vi "DCDC_Command.vi"(8 "error in (no error)":errorcluster, 9 "State":bool, 10 "Function Choose":T1, 11 "VISA resource in":refnum<visa-resource-name>="COM9") -> (0 "error out":errorcluster, 1 "Result":bool, 2 "read buffer":string, 3 "VISA resource out":refnum<visa-resource-name>)   [LabVIEW 2020]
uses:
  subvi/DCDC_Command.ctl
  ed6a49d5-09bc-4943-8c1b-6836990d678a.vi
  932ad59c-eb7e-44d9-8b1f-b581c4131119.vi
  c181c2eb-5caa-41f7-8f1d-9b0969fe7b32.vi
  9037c64f-12a5-4f95-b925-5e25449c8f50.vi
  f13df80e-a96c-4ee4-8010-69a0a001d2db.vi
  470163fb-24ed-4801-9874-fb3a4beeb085.vi
  c287b82f-2120-49b1-88be-16a92ee30e73.vi
  f2adf25f-970b-415f-a032-e0fcf203b769.vi
  9be719b3-8aa6-4acf-ac95-30d0a9685e01.vi
  5b62b920-1295-4d0c-95f0-4be6a500b32e.vi
  654ba534-6598-400c-ba18-c9c01572c5a6.vi
  4029cff3-6ee8-466a-8162-b4f2fed149be.vi
  8d00504a-0fe9-4555-a6c6-77f6f728d10d.vi
  74fb5378-ac97-4efc-aca6-68fbee075285.vi
  491523d6-905e-4462-ba80-ce53b186b227.vi
  b9b75ff8-5319-4f28-8b4f-30b6a65af060.vi
  a2ce7b80-4b4e-4363-a8f0-59d5445ac21a.vi
  c57a13a5-17d0-45dd-b178-92708c13f94c.vi
  b9cf9fe5-3c0b-4bbf-9f32-9392ab34740f.vi
  d481e0cc-f03c-4cb3-989f-8431de273cff.vi
  7cc232e6-0bf6-4d56-8fbd-2d34dd7a08cb.vi
  4c5eb965-6c60-44f3-beb1-d14c2485ea10.vi
  9afb1382-b455-4c0e-a240-fdb1f9a06be5.vi
  cd49513f-002c-4f77-9f81-ccd1a5219046.vi
  d0cc9776-c1ff-4c24-bdcf-5ded2007c62b.vi
  86a8435c-e44f-4f7e-af84-550518831f96.vi
  b69966e4-5735-4af5-b3a8-09b30bbeab7e.vi
  00024ba3-8fb2-44c0-bc84-52fe597d7133.vi
  584b1e2f-3a49-4222-b9e3-bc359bacf4d8.vi
  dfd3edac-81af-4fc9-8c20-3b86a2300b8a.vi
  99b15c50-76b8-4825-9a13-4551792e8dd0.vi
  55bbcbfe-8e8e-49d6-aef4-1d5580b9a963.vi
  beff6438-17f9-41f9-9810-ebce5ae72097.vi
  f2b4e730-93e4-4862-a775-5e8cbcdf507d.vi
  446e0732-4c03-44b1-82af-2731cf1dbfa6.vi
  5ef83345-9fb9-4ebf-ae3d-3223e83d8c37.vi
  b02090d9-b192-45ba-be58-8757ebd68618.vi
  1e0aad6e-494a-45e0-8f3c-aae04b02fd79.vi
  27daadd7-8e79-41ca-a841-e16ae762918d.vi
  4dcf7d4f-3f4f-43d3-8a35-0787c73001a8.vi
  43c5c4f2-1bb4-495d-bee3-a4e32fcfdcb9.vi
  4b4ab4a6-5e5d-45c8-b5c7-9b4ed80b424c.vi
  3a2d3712-2a36-4ec5-9aeb-46b5983d2c7c.vi
  54e5a227-360d-442c-a17c-3ce3fac416c0.vi
  26761caf-5a13-4f0c-bc23-988e0c337ddd.vi
  bcf161b8-5927-4e65-bc1d-9e8474243abe.vi
  404ad2bd-238a-4596-8c97-1917f7eafb42.vi
  7b1b14b6-a11a-4e71-b5fe-a22ca238d731.vi
  cc6ea0eb-ab18-458c-8049-5ca8eac1973d.vi
  4ab0fb06-892c-4162-8198-9fc52b03e3cd.vi
  6f6dd622-ab08-4417-a5cc-d92aaecab5e4.vi
  819ae6c1-48a2-4b0c-aee5-2a930aacc770.vi
  6b5f23c1-0d39-4d1f-9992-30a1b69dbdde.vi
  a3966776-c575-48a1-b1d1-d3cf2a5ccec7.vi
  dc90b0fe-1ec9-40c7-8bd3-7877db3c712c.vi
  <vilib>/Instr/_visa.llb/VISA Configure Serial Port (Instr).vi
panel:
  # "Board1_ll1"
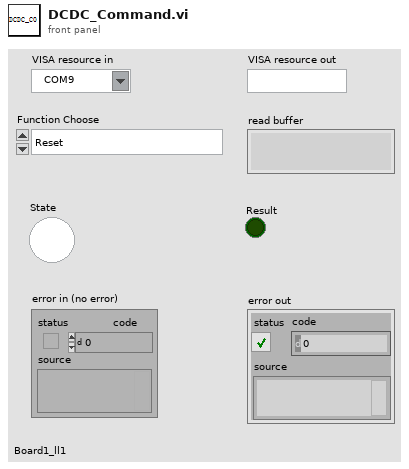
[diagram p1: front panel]
types:
  T1 = typedef "DCDC_Command.ctl" = enum16{"Reset", "APOS_SENSE", "ANEG_SENSE", "DPOS_SENSE", "FCT_SW1", "FCT_SW2", "FCT_SW3", "ANEG_LOAD", "APOS_LOAD", "DPOS_LOAD", "Short ANEG", "Short APOS", "Short DPOS", "meas_PSU_1_12V", "meas_PSU_2_12V", "meas_PSU_3_12V", "meas_UUT_APOS_voltage", "meas_UUT_ANEG_voltage", "meas_UUT_DPOS_voltage", "meas_LOAD_APOS_voltage", "meas_LOAD_ANEG_voltage", "meas_LOAD_DPOS_voltage", "UUT_FCT_power_SW", "Burn_in_FAN_SW", "FCT_FAN_SW", "FCT_24V_SW", "USB_Reset", "DMM_SW"}
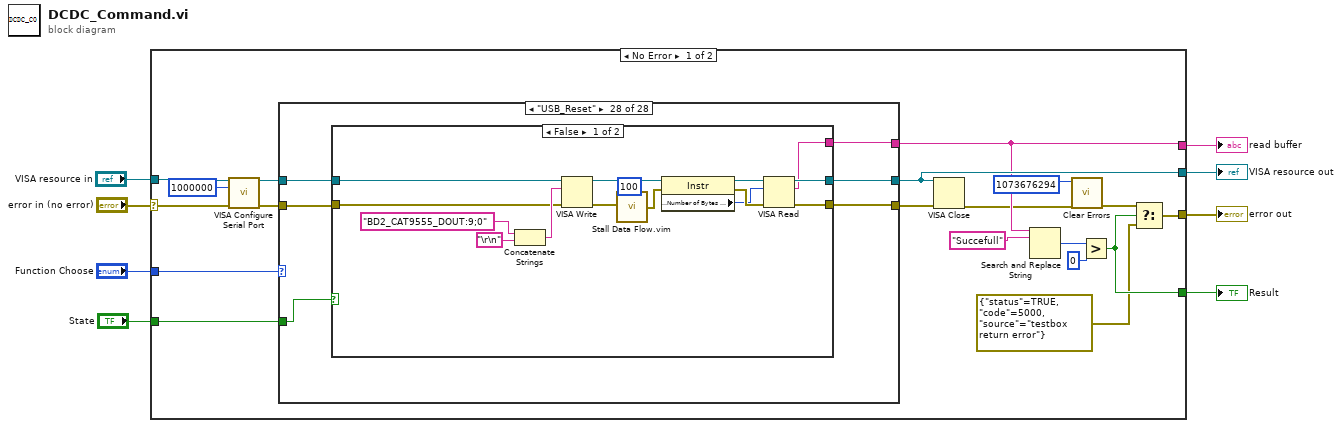
[diagram p0: block diagram]
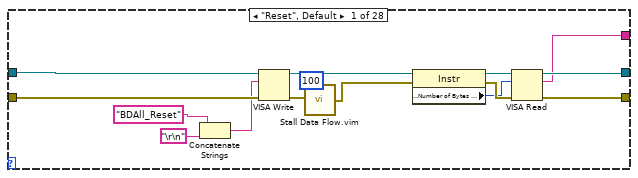
[diagram p2: hidden frame]
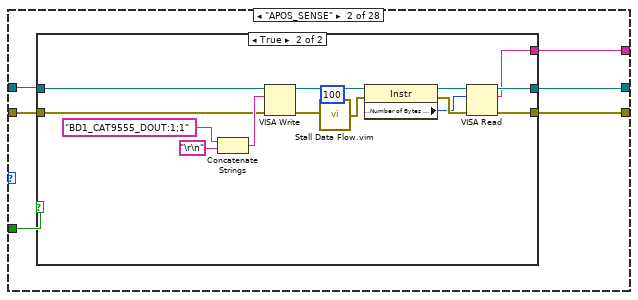
[diagram p3: hidden frame]
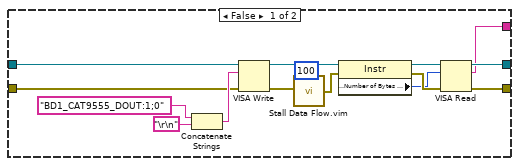
[diagram p4: hidden frame]
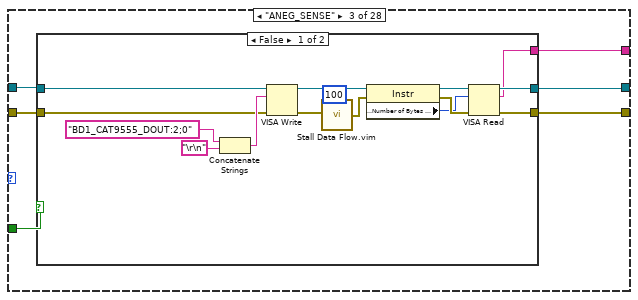
[diagram p5: hidden frame]
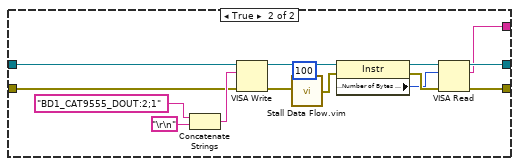
[diagram p6: hidden frame]
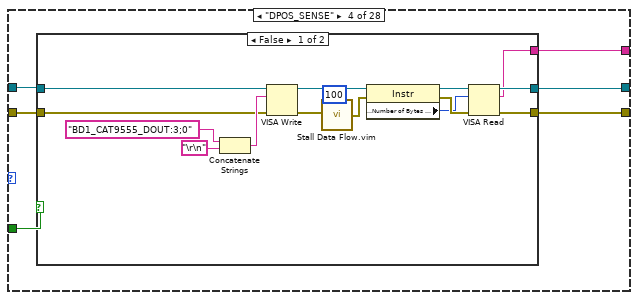
[diagram p7: hidden frame]
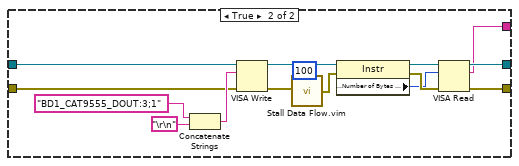
[diagram p8: hidden frame]
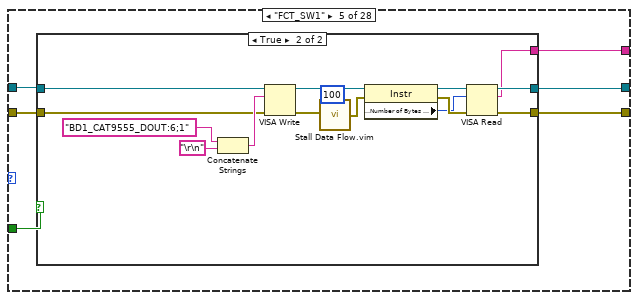
[diagram p9: hidden frame]
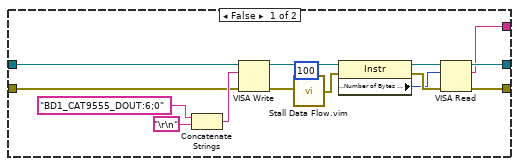
[diagram p10: hidden frame]
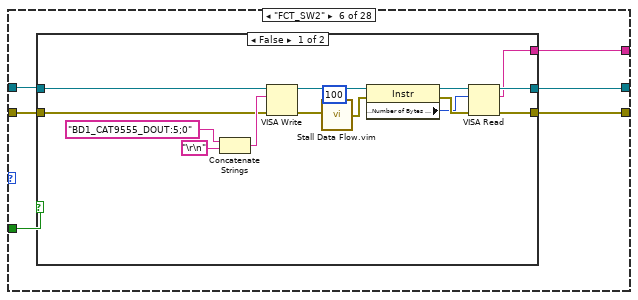
[diagram p11: hidden frame]
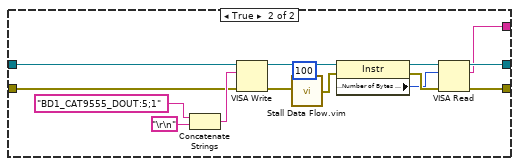
[diagram p12: hidden frame]
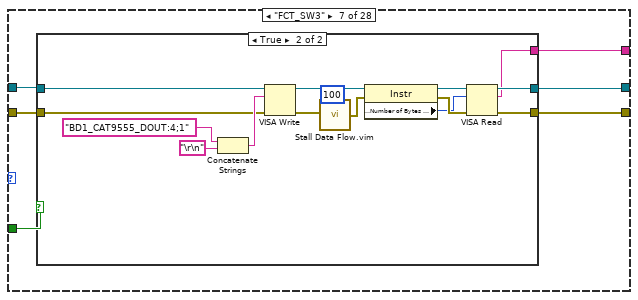
[diagram p13: hidden frame]
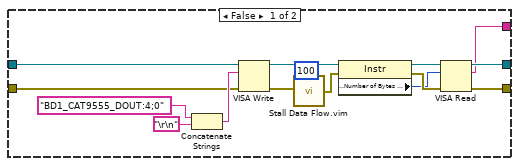
[diagram p14: hidden frame]
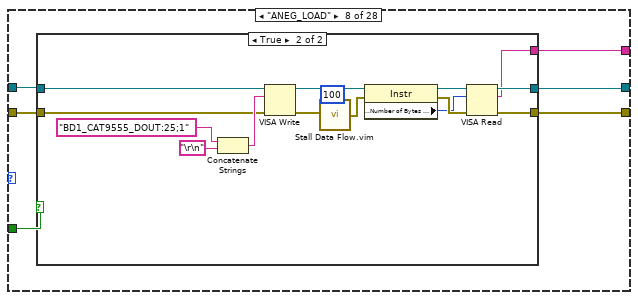
[diagram p15: hidden frame]
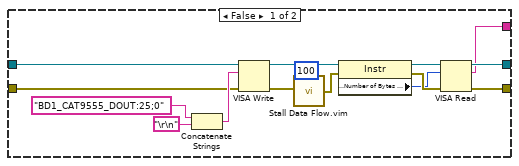
[diagram p16: hidden frame]
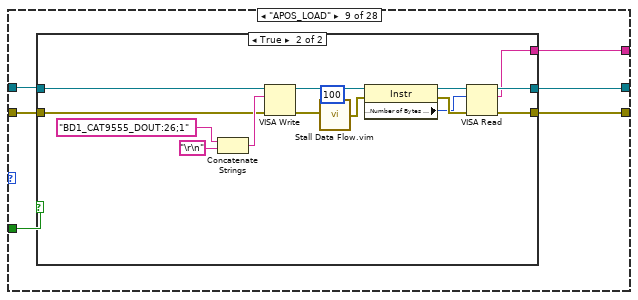
[diagram p17: hidden frame]
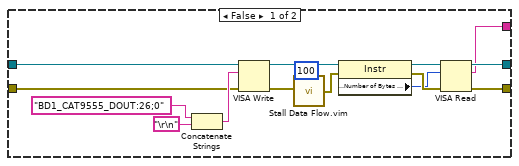
[diagram p18: hidden frame]
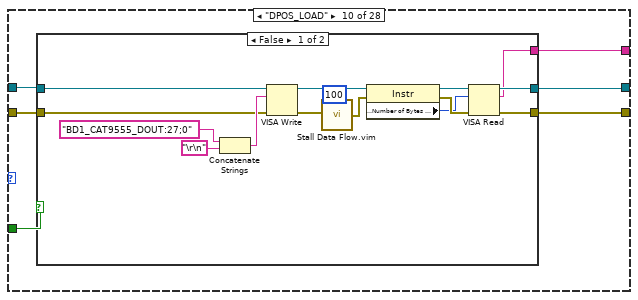
[diagram p19: hidden frame]
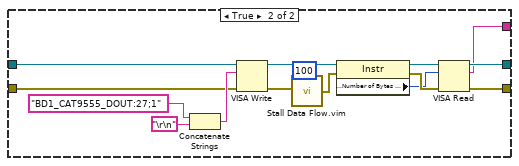
[diagram p20: hidden frame]
diagram:
  n1 = case shown="No Error" "error in (no error)" {
    selector: "error in (no error)" -> [w23 w1025]
    tunnel: "Function Choose" -> [w27 _]
    tunnel: "State" -> [w26 _]
    tunnel: "VISA resource in" -> [w24 _]
    tunnel: [w20 _] -> w4
    tunnel: [w19 _] -> w3
    tunnel: [w12 _] -> w2
    tunnel: [w10 w1025] -> w1
    frame No Error {
      n2 = call-poly "VISA Configure Serial Port"("VISA resource name"=w24, "baud rate (9600)"=u32 1000000, "error in (no error)"=w23) -> ("VISA resource name out"=w25:refnum<visa-resource-name>, "error out"=w22:errorcluster)  [unwired: 11 in]
      n3 = case shown="\"USB_Reset\"" w27 {
        tunnel: w26 -> [_ w46 w82 w118 w154 w190 w226 w262 w298 w334 w370 w406 w442 w478 w514 w550 w586 w622 w658 w694 w730 w766 w802 w838 w874 w910 w946 w992]
        tunnel: w25 -> [w41 w48 w84 w120 w156 w192 w228 w264 w300 w336 w372 w408 w444 w480 w516 w552 w588 w624 w660 w696 w732 w768 w804 w840 w876 w912 w948 w993]
        tunnel: w22 -> [w42 w47 w83 w119 w155 w191 w227 w263 w299 w335 w371 w407 w443 w479 w515 w551 w587 w623 w659 w695 w731 w767 w803 w839 w875 w911 w947 w994]
        tunnel: [w39 w45 w81 w117 w153 w189 w225 w261 w297 w333 w369 w405 w441 w477 w513 w549 w585 w621 w657 w693 w729 w765 w801 w837 w871 w909 w945 w991] -> w21
        tunnel: [w40 w44 w80 w116 w152 w188 w224 w260 w296 w332 w368 w404 w440 w476 w512 w548 w584 w620 w656 w692 w728 w764 w800 w836 w872 w908 w944 w990] -> w20
        tunnel: [w34 w43 w79 w115 w151 w187 w223 w259 w295 w331 w367 w403 w439 w475 w511 w547 w583 w619 w655 w691 w727 w763 w799 w835 w873 w907 w943 w989] -> w19
        frame "Reset", Default {
          n4 = Concatenate Strings("BDAll_Reset" ("write buffer"), "\r\n") -> (w31:string)
          n5 = VISA Write(VISA resource name=w41, write buffer=w31, error in (no error)=w42) -> (VISA resource name out=w38:refnum<visa-resource-name>, error out=w30:errorcluster)  [unwired: 1 out]
          n6 = call "Stall Data Flow.vim"("value in"=w30, "milliseconds to wait"=u32 100) -> ("value out"=w29:errorcluster)  [unwired: 1 out]
          n7 = property class="Instr"(reference=w38, error in=w29) -> (reference out=w37:refnum<visa-resource-name>, error out=w36:errorcluster, "Serial Settings:Number of Bytes at Serial Port"=w35:u32)
          n8 = VISA Read(VISA resource name=w37, byte count=w35, error in (no error)=w36) -> (VISA resource name out=w40:refnum<visa-resource-name>, read buffer=w34:string, error out=w39:errorcluster)  [unwired: 1 out]
        }
        frame "APOS_SENSE" {
          n9 = case shown="True" w46 {
            tunnel: w48 -> [w54 w69]
            tunnel: w47 -> [w53 w68]
            tunnel: [w52 w66] -> w45
            tunnel: [w51 w67] -> w44
            tunnel: [w50 w65] -> w43
            frame False {
              n10 = Concatenate Strings("BD1_CAT9555_DOUT:1;0" ("write buffer"), "\r\n") -> (w58:string)
              n11 = VISA Write(VISA resource name=w54, write buffer=w58, error in (no error)=w53) -> (VISA resource name out=w63:refnum<visa-resource-name>, error out=w57:errorcluster)  [unwired: 1 out]
              n12 = call "Stall Data Flow.vim"("value in"=w57, "milliseconds to wait"=u32 100) -> ("value out"=w56:errorcluster)  [unwired: 1 out]
              n13 = property class="Instr"(reference=w63, error in=w56) -> (reference out=w62:refnum<visa-resource-name>, error out=w61:errorcluster, "Serial Settings:Number of Bytes at Serial Port"=w60:u32)
              n14 = VISA Read(VISA resource name=w62, byte count=w60, error in (no error)=w61) -> (VISA resource name out=w51:refnum<visa-resource-name>, read buffer=w50:string, error out=w52:errorcluster)  [unwired: 1 out]
            }
            frame True {
              n15 = Concatenate Strings("BD1_CAT9555_DOUT:1;1" ("write buffer"), "\r\n") -> (w73:string)
              n16 = VISA Write(VISA resource name=w69, write buffer=w73, error in (no error)=w68) -> (VISA resource name out=w78:refnum<visa-resource-name>, error out=w72:errorcluster)  [unwired: 1 out]
              n17 = call "Stall Data Flow.vim"("value in"=w72, "milliseconds to wait"=u32 100) -> ("value out"=w71:errorcluster)  [unwired: 1 out]
              n18 = property class="Instr"(reference=w78, error in=w71) -> (reference out=w77:refnum<visa-resource-name>, error out=w76:errorcluster, "Serial Settings:Number of Bytes at Serial Port"=w75:u32)
              n19 = VISA Read(VISA resource name=w77, byte count=w75, error in (no error)=w76) -> (VISA resource name out=w67:refnum<visa-resource-name>, read buffer=w65:string, error out=w66:errorcluster)  [unwired: 1 out]
            }
          }
        }
        frame "ANEG_SENSE" {
          n20 = case shown="False" w82 {
            tunnel: w84 -> [w90 w105]
            tunnel: w83 -> [w89 w104]
            tunnel: [w88 w102] -> w81
            tunnel: [w87 w103] -> w80
            tunnel: [w86 w101] -> w79
            frame False {
              n21 = Concatenate Strings("BD1_CAT9555_DOUT:2;0" ("write buffer"), "\r\n") -> (w94:string)
              n22 = VISA Write(VISA resource name=w90, write buffer=w94, error in (no error)=w89) -> (VISA resource name out=w99:refnum<visa-resource-name>, error out=w93:errorcluster)  [unwired: 1 out]
              n23 = call "Stall Data Flow.vim"("value in"=w93, "milliseconds to wait"=u32 100) -> ("value out"=w92:errorcluster)  [unwired: 1 out]
              n24 = property class="Instr"(reference=w99, error in=w92) -> (reference out=w98:refnum<visa-resource-name>, error out=w97:errorcluster, "Serial Settings:Number of Bytes at Serial Port"=w96:u32)
              n25 = VISA Read(VISA resource name=w98, byte count=w96, error in (no error)=w97) -> (VISA resource name out=w87:refnum<visa-resource-name>, read buffer=w86:string, error out=w88:errorcluster)  [unwired: 1 out]
            }
            frame True {
              n26 = Concatenate Strings("BD1_CAT9555_DOUT:2;1" ("write buffer"), "\r\n") -> (w109:string)
              n27 = VISA Write(VISA resource name=w105, write buffer=w109, error in (no error)=w104) -> (VISA resource name out=w114:refnum<visa-resource-name>, error out=w108:errorcluster)  [unwired: 1 out]
              n28 = call "Stall Data Flow.vim"("value in"=w108, "milliseconds to wait"=u32 100) -> ("value out"=w107:errorcluster)  [unwired: 1 out]
              n29 = property class="Instr"(reference=w114, error in=w107) -> (reference out=w113:refnum<visa-resource-name>, error out=w112:errorcluster, "Serial Settings:Number of Bytes at Serial Port"=w111:u32)
              n30 = VISA Read(VISA resource name=w113, byte count=w111, error in (no error)=w112) -> (VISA resource name out=w103:refnum<visa-resource-name>, read buffer=w101:string, error out=w102:errorcluster)  [unwired: 1 out]
            }
          }
        }
        frame "DPOS_SENSE" {
          n31 = case shown="False" w118 {
            tunnel: w120 -> [w126 w141]
            tunnel: w119 -> [w125 w140]
            tunnel: [w124 w138] -> w117
            tunnel: [w123 w139] -> w116
            tunnel: [w122 w137] -> w115
            frame False {
              n32 = Concatenate Strings("BD1_CAT9555_DOUT:3;0" ("write buffer"), "\r\n") -> (w130:string)
              n33 = VISA Write(VISA resource name=w126, write buffer=w130, error in (no error)=w125) -> (VISA resource name out=w135:refnum<visa-resource-name>, error out=w129:errorcluster)  [unwired: 1 out]
              n34 = call "Stall Data Flow.vim"("value in"=w129, "milliseconds to wait"=u32 100) -> ("value out"=w128:errorcluster)  [unwired: 1 out]
              n35 = property class="Instr"(reference=w135, error in=w128) -> (reference out=w134:refnum<visa-resource-name>, error out=w133:errorcluster, "Serial Settings:Number of Bytes at Serial Port"=w132:u32)
              n36 = VISA Read(VISA resource name=w134, byte count=w132, error in (no error)=w133) -> (VISA resource name out=w123:refnum<visa-resource-name>, read buffer=w122:string, error out=w124:errorcluster)  [unwired: 1 out]
            }
            frame True {
              n37 = Concatenate Strings("BD1_CAT9555_DOUT:3;1" ("write buffer"), "\r\n") -> (w145:string)
              n38 = VISA Write(VISA resource name=w141, write buffer=w145, error in (no error)=w140) -> (VISA resource name out=w150:refnum<visa-resource-name>, error out=w144:errorcluster)  [unwired: 1 out]
              n39 = call "Stall Data Flow.vim"("value in"=w144, "milliseconds to wait"=u32 100) -> ("value out"=w143:errorcluster)  [unwired: 1 out]
              n40 = property class="Instr"(reference=w150, error in=w143) -> (reference out=w149:refnum<visa-resource-name>, error out=w148:errorcluster, "Serial Settings:Number of Bytes at Serial Port"=w147:u32)
              n41 = VISA Read(VISA resource name=w149, byte count=w147, error in (no error)=w148) -> (VISA resource name out=w139:refnum<visa-resource-name>, read buffer=w137:string, error out=w138:errorcluster)  [unwired: 1 out]
            }
          }
        }
        frame "FCT_SW1" {
          n42 = case shown="True" w154 {
            tunnel: w156 -> [w162 w177]
            tunnel: w155 -> [w161 w176]
            tunnel: [w160 w174] -> w153
            tunnel: [w159 w175] -> w152
            tunnel: [w158 w173] -> w151
            frame False {
              n43 = Concatenate Strings("BD1_CAT9555_DOUT:6;0" ("write buffer"), "\r\n") -> (w166:string)
              n44 = VISA Write(VISA resource name=w162, write buffer=w166, error in (no error)=w161) -> (VISA resource name out=w171:refnum<visa-resource-name>, error out=w165:errorcluster)  [unwired: 1 out]
              n45 = call "Stall Data Flow.vim"("value in"=w165, "milliseconds to wait"=u32 100) -> ("value out"=w164:errorcluster)  [unwired: 1 out]
              n46 = property class="Instr"(reference=w171, error in=w164) -> (reference out=w170:refnum<visa-resource-name>, error out=w169:errorcluster, "Serial Settings:Number of Bytes at Serial Port"=w168:u32)
              n47 = VISA Read(VISA resource name=w170, byte count=w168, error in (no error)=w169) -> (VISA resource name out=w159:refnum<visa-resource-name>, read buffer=w158:string, error out=w160:errorcluster)  [unwired: 1 out]
            }
            frame True {
              n48 = Concatenate Strings("BD1_CAT9555_DOUT:6;1" ("write buffer"), "\r\n") -> (w181:string)
              n49 = VISA Write(VISA resource name=w177, write buffer=w181, error in (no error)=w176) -> (VISA resource name out=w186:refnum<visa-resource-name>, error out=w180:errorcluster)  [unwired: 1 out]
              n50 = call "Stall Data Flow.vim"("value in"=w180, "milliseconds to wait"=u32 100) -> ("value out"=w179:errorcluster)  [unwired: 1 out]
              n51 = property class="Instr"(reference=w186, error in=w179) -> (reference out=w185:refnum<visa-resource-name>, error out=w184:errorcluster, "Serial Settings:Number of Bytes at Serial Port"=w183:u32)
              n52 = VISA Read(VISA resource name=w185, byte count=w183, error in (no error)=w184) -> (VISA resource name out=w175:refnum<visa-resource-name>, read buffer=w173:string, error out=w174:errorcluster)  [unwired: 1 out]
            }
          }
        }
        frame "FCT_SW2" {
          n53 = case shown="False" w190 {
            tunnel: w192 -> [w198 w213]
            tunnel: w191 -> [w197 w212]
            tunnel: [w196 w210] -> w189
            tunnel: [w195 w211] -> w188
            tunnel: [w194 w209] -> w187
            frame False {
              n54 = Concatenate Strings("BD1_CAT9555_DOUT:5;0" ("write buffer"), "\r\n") -> (w202:string)
              n55 = VISA Write(VISA resource name=w198, write buffer=w202, error in (no error)=w197) -> (VISA resource name out=w207:refnum<visa-resource-name>, error out=w201:errorcluster)  [unwired: 1 out]
              n56 = call "Stall Data Flow.vim"("value in"=w201, "milliseconds to wait"=u32 100) -> ("value out"=w200:errorcluster)  [unwired: 1 out]
              n57 = property class="Instr"(reference=w207, error in=w200) -> (reference out=w206:refnum<visa-resource-name>, error out=w205:errorcluster, "Serial Settings:Number of Bytes at Serial Port"=w204:u32)
              n58 = VISA Read(VISA resource name=w206, byte count=w204, error in (no error)=w205) -> (VISA resource name out=w195:refnum<visa-resource-name>, read buffer=w194:string, error out=w196:errorcluster)  [unwired: 1 out]
            }
            frame True {
              n59 = Concatenate Strings("BD1_CAT9555_DOUT:5;1" ("write buffer"), "\r\n") -> (w217:string)
              n60 = VISA Write(VISA resource name=w213, write buffer=w217, error in (no error)=w212) -> (VISA resource name out=w222:refnum<visa-resource-name>, error out=w216:errorcluster)  [unwired: 1 out]
              n61 = call "Stall Data Flow.vim"("value in"=w216, "milliseconds to wait"=u32 100) -> ("value out"=w215:errorcluster)  [unwired: 1 out]
              n62 = property class="Instr"(reference=w222, error in=w215) -> (reference out=w221:refnum<visa-resource-name>, error out=w220:errorcluster, "Serial Settings:Number of Bytes at Serial Port"=w219:u32)
              n63 = VISA Read(VISA resource name=w221, byte count=w219, error in (no error)=w220) -> (VISA resource name out=w211:refnum<visa-resource-name>, read buffer=w209:string, error out=w210:errorcluster)  [unwired: 1 out]
            }
          }
        }
        frame "FCT_SW3" {
          n64 = case shown="True" w226 {
            tunnel: w228 -> [w234 w249]
            tunnel: w227 -> [w233 w248]
            tunnel: [w232 w246] -> w225
            tunnel: [w231 w247] -> w224
            tunnel: [w230 w245] -> w223
            frame False {
              n65 = Concatenate Strings("BD1_CAT9555_DOUT:4;0" ("write buffer"), "\r\n") -> (w238:string)
              n66 = VISA Write(VISA resource name=w234, write buffer=w238, error in (no error)=w233) -> (VISA resource name out=w243:refnum<visa-resource-name>, error out=w237:errorcluster)  [unwired: 1 out]
              n67 = call "Stall Data Flow.vim"("value in"=w237, "milliseconds to wait"=u32 100) -> ("value out"=w236:errorcluster)  [unwired: 1 out]
              n68 = property class="Instr"(reference=w243, error in=w236) -> (reference out=w242:refnum<visa-resource-name>, error out=w241:errorcluster, "Serial Settings:Number of Bytes at Serial Port"=w240:u32)
              n69 = VISA Read(VISA resource name=w242, byte count=w240, error in (no error)=w241) -> (VISA resource name out=w231:refnum<visa-resource-name>, read buffer=w230:string, error out=w232:errorcluster)  [unwired: 1 out]
            }
            frame True {
              n70 = Concatenate Strings("BD1_CAT9555_DOUT:4;1" ("write buffer"), "\r\n") -> (w253:string)
              n71 = VISA Write(VISA resource name=w249, write buffer=w253, error in (no error)=w248) -> (VISA resource name out=w258:refnum<visa-resource-name>, error out=w252:errorcluster)  [unwired: 1 out]
              n72 = call "Stall Data Flow.vim"("value in"=w252, "milliseconds to wait"=u32 100) -> ("value out"=w251:errorcluster)  [unwired: 1 out]
              n73 = property class="Instr"(reference=w258, error in=w251) -> (reference out=w257:refnum<visa-resource-name>, error out=w256:errorcluster, "Serial Settings:Number of Bytes at Serial Port"=w255:u32)
              n74 = VISA Read(VISA resource name=w257, byte count=w255, error in (no error)=w256) -> (VISA resource name out=w247:refnum<visa-resource-name>, read buffer=w245:string, error out=w246:errorcluster)  [unwired: 1 out]
            }
          }
        }
        frame "ANEG_LOAD" {
          n75 = case shown="True" w262 {
            tunnel: w264 -> [w270 w285]
            tunnel: w263 -> [w269 w284]
            tunnel: [w268 w282] -> w261
            tunnel: [w267 w283] -> w260
            tunnel: [w266 w281] -> w259
            frame False {
              n76 = Concatenate Strings("BD1_CAT9555_DOUT:25;0" ("write buffer"), "\r\n") -> (w274:string)
              n77 = VISA Write(VISA resource name=w270, write buffer=w274, error in (no error)=w269) -> (VISA resource name out=w279:refnum<visa-resource-name>, error out=w273:errorcluster)  [unwired: 1 out]
              n78 = call "Stall Data Flow.vim"("value in"=w273, "milliseconds to wait"=u32 100) -> ("value out"=w272:errorcluster)  [unwired: 1 out]
              n79 = property class="Instr"(reference=w279, error in=w272) -> (reference out=w278:refnum<visa-resource-name>, error out=w277:errorcluster, "Serial Settings:Number of Bytes at Serial Port"=w276:u32)
              n80 = VISA Read(VISA resource name=w278, byte count=w276, error in (no error)=w277) -> (VISA resource name out=w267:refnum<visa-resource-name>, read buffer=w266:string, error out=w268:errorcluster)  [unwired: 1 out]
            }
            frame True {
              n81 = Concatenate Strings("BD1_CAT9555_DOUT:25;1" ("write buffer"), "\r\n") -> (w289:string)
              n82 = VISA Write(VISA resource name=w285, write buffer=w289, error in (no error)=w284) -> (VISA resource name out=w294:refnum<visa-resource-name>, error out=w288:errorcluster)  [unwired: 1 out]
              n83 = call "Stall Data Flow.vim"("value in"=w288, "milliseconds to wait"=u32 100) -> ("value out"=w287:errorcluster)  [unwired: 1 out]
              n84 = property class="Instr"(reference=w294, error in=w287) -> (reference out=w293:refnum<visa-resource-name>, error out=w292:errorcluster, "Serial Settings:Number of Bytes at Serial Port"=w291:u32)
              n85 = VISA Read(VISA resource name=w293, byte count=w291, error in (no error)=w292) -> (VISA resource name out=w283:refnum<visa-resource-name>, read buffer=w281:string, error out=w282:errorcluster)  [unwired: 1 out]
            }
          }
        }
        frame "APOS_LOAD" {
          n86 = case shown="True" w298 {
            tunnel: w300 -> [w306 w321]
            tunnel: w299 -> [w305 w320]
            tunnel: [w304 w318] -> w297
            tunnel: [w303 w319] -> w296
            tunnel: [w302 w317] -> w295
            frame False {
              n87 = Concatenate Strings("BD1_CAT9555_DOUT:26;0" ("write buffer"), "\r\n") -> (w310:string)
              n88 = VISA Write(VISA resource name=w306, write buffer=w310, error in (no error)=w305) -> (VISA resource name out=w315:refnum<visa-resource-name>, error out=w309:errorcluster)  [unwired: 1 out]
              n89 = call "Stall Data Flow.vim"("value in"=w309, "milliseconds to wait"=u32 100) -> ("value out"=w308:errorcluster)  [unwired: 1 out]
              n90 = property class="Instr"(reference=w315, error in=w308) -> (reference out=w314:refnum<visa-resource-name>, error out=w313:errorcluster, "Serial Settings:Number of Bytes at Serial Port"=w312:u32)
              n91 = VISA Read(VISA resource name=w314, byte count=w312, error in (no error)=w313) -> (VISA resource name out=w303:refnum<visa-resource-name>, read buffer=w302:string, error out=w304:errorcluster)  [unwired: 1 out]
            }
            frame True {
              n92 = Concatenate Strings("BD1_CAT9555_DOUT:26;1" ("write buffer"), "\r\n") -> (w325:string)
              n93 = VISA Write(VISA resource name=w321, write buffer=w325, error in (no error)=w320) -> (VISA resource name out=w330:refnum<visa-resource-name>, error out=w324:errorcluster)  [unwired: 1 out]
              n94 = call "Stall Data Flow.vim"("value in"=w324, "milliseconds to wait"=u32 100) -> ("value out"=w323:errorcluster)  [unwired: 1 out]
              n95 = property class="Instr"(reference=w330, error in=w323) -> (reference out=w329:refnum<visa-resource-name>, error out=w328:errorcluster, "Serial Settings:Number of Bytes at Serial Port"=w327:u32)
              n96 = VISA Read(VISA resource name=w329, byte count=w327, error in (no error)=w328) -> (VISA resource name out=w319:refnum<visa-resource-name>, read buffer=w317:string, error out=w318:errorcluster)  [unwired: 1 out]
            }
          }
        }
        frame "DPOS_LOAD" {
          n97 = case shown="False" w334 {
            tunnel: w336 -> [w342 w357]
            tunnel: w335 -> [w341 w356]
            tunnel: [w340 w354] -> w333
            tunnel: [w339 w355] -> w332
            tunnel: [w338 w353] -> w331
            frame False {
              n98 = Concatenate Strings("BD1_CAT9555_DOUT:27;0" ("write buffer"), "\r\n") -> (w346:string)
              n99 = VISA Write(VISA resource name=w342, write buffer=w346, error in (no error)=w341) -> (VISA resource name out=w351:refnum<visa-resource-name>, error out=w345:errorcluster)  [unwired: 1 out]
              n100 = call "Stall Data Flow.vim"("value in"=w345, "milliseconds to wait"=u32 100) -> ("value out"=w344:errorcluster)  [unwired: 1 out]
              n101 = property class="Instr"(reference=w351, error in=w344) -> (reference out=w350:refnum<visa-resource-name>, error out=w349:errorcluster, "Serial Settings:Number of Bytes at Serial Port"=w348:u32)
              n102 = VISA Read(VISA resource name=w350, byte count=w348, error in (no error)=w349) -> (VISA resource name out=w339:refnum<visa-resource-name>, read buffer=w338:string, error out=w340:errorcluster)  [unwired: 1 out]
            }
            frame True {
              n103 = Concatenate Strings("BD1_CAT9555_DOUT:27;1" ("write buffer"), "\r\n") -> (w361:string)
              n104 = VISA Write(VISA resource name=w357, write buffer=w361, error in (no error)=w356) -> (VISA resource name out=w366:refnum<visa-resource-name>, error out=w360:errorcluster)  [unwired: 1 out]
              n105 = call "Stall Data Flow.vim"("value in"=w360, "milliseconds to wait"=u32 100) -> ("value out"=w359:errorcluster)  [unwired: 1 out]
              n106 = property class="Instr"(reference=w366, error in=w359) -> (reference out=w365:refnum<visa-resource-name>, error out=w364:errorcluster, "Serial Settings:Number of Bytes at Serial Port"=w363:u32)
              n107 = VISA Read(VISA resource name=w365, byte count=w363, error in (no error)=w364) -> (VISA resource name out=w355:refnum<visa-resource-name>, read buffer=w353:string, error out=w354:errorcluster)  [unwired: 1 out]
            }
          }
        }
        frame "Short ANEG" {
          n108 = case shown="True" w370 {
            tunnel: w372 -> [w378 w393]
            tunnel: w371 -> [w377 w392]
            tunnel: [w376 w390] -> w369
            tunnel: [w375 w391] -> w368
            tunnel: [w374 w389] -> w367
            frame False {
              n109 = Concatenate Strings("BD1_CAT9555_DOUT:28;0" ("write buffer"), "\r\n") -> (w382:string)
              n110 = VISA Write(VISA resource name=w378, write buffer=w382, error in (no error)=w377) -> (VISA resource name out=w387:refnum<visa-resource-name>, error out=w381:errorcluster)  [unwired: 1 out]
              n111 = call "Stall Data Flow.vim"("value in"=w381, "milliseconds to wait"=u32 100) -> ("value out"=w380:errorcluster)  [unwired: 1 out]
              n112 = property class="Instr"(reference=w387, error in=w380) -> (reference out=w386:refnum<visa-resource-name>, error out=w385:errorcluster, "Serial Settings:Number of Bytes at Serial Port"=w384:u32)
              n113 = VISA Read(VISA resource name=w386, byte count=w384, error in (no error)=w385) -> (VISA resource name out=w375:refnum<visa-resource-name>, read buffer=w374:string, error out=w376:errorcluster)  [unwired: 1 out]
            }
            frame True {
              n114 = Concatenate Strings("BD1_CAT9555_DOUT:28;1" ("write buffer"), "\r\n") -> (w397:string)
              n115 = VISA Write(VISA resource name=w393, write buffer=w397, error in (no error)=w392) -> (VISA resource name out=w402:refnum<visa-resource-name>, error out=w396:errorcluster)  [unwired: 1 out]
              n116 = call "Stall Data Flow.vim"("value in"=w396, "milliseconds to wait"=u32 100) -> ("value out"=w395:errorcluster)  [unwired: 1 out]
              n117 = property class="Instr"(reference=w402, error in=w395) -> (reference out=w401:refnum<visa-resource-name>, error out=w400:errorcluster, "Serial Settings:Number of Bytes at Serial Port"=w399:u32)
              n118 = VISA Read(VISA resource name=w401, byte count=w399, error in (no error)=w400) -> (VISA resource name out=w391:refnum<visa-resource-name>, read buffer=w389:string, error out=w390:errorcluster)  [unwired: 1 out]
            }
          }
        }
        frame "Short APOS" {
          n119 = case shown="False" w406 {
            tunnel: w408 -> [w414 w429]
            tunnel: w407 -> [w413 w428]
            tunnel: [w412 w426] -> w405
            tunnel: [w411 w427] -> w404
            tunnel: [w410 w425] -> w403
            frame False {
              n120 = Concatenate Strings("BD1_CAT9555_DOUT:29;0" ("write buffer"), "\r\n") -> (w418:string)
              n121 = VISA Write(VISA resource name=w414, write buffer=w418, error in (no error)=w413) -> (VISA resource name out=w423:refnum<visa-resource-name>, error out=w417:errorcluster)  [unwired: 1 out]
              n122 = call "Stall Data Flow.vim"("value in"=w417, "milliseconds to wait"=u32 100) -> ("value out"=w416:errorcluster)  [unwired: 1 out]
              n123 = property class="Instr"(reference=w423, error in=w416) -> (reference out=w422:refnum<visa-resource-name>, error out=w421:errorcluster, "Serial Settings:Number of Bytes at Serial Port"=w420:u32)
              n124 = VISA Read(VISA resource name=w422, byte count=w420, error in (no error)=w421) -> (VISA resource name out=w411:refnum<visa-resource-name>, read buffer=w410:string, error out=w412:errorcluster)  [unwired: 1 out]
            }
            frame True {
              n125 = Concatenate Strings("BD1_CAT9555_DOUT:29;1" ("write buffer"), "\r\n") -> (w433:string)
              n126 = VISA Write(VISA resource name=w429, write buffer=w433, error in (no error)=w428) -> (VISA resource name out=w438:refnum<visa-resource-name>, error out=w432:errorcluster)  [unwired: 1 out]
              n127 = call "Stall Data Flow.vim"("value in"=w432, "milliseconds to wait"=u32 100) -> ("value out"=w431:errorcluster)  [unwired: 1 out]
              n128 = property class="Instr"(reference=w438, error in=w431) -> (reference out=w437:refnum<visa-resource-name>, error out=w436:errorcluster, "Serial Settings:Number of Bytes at Serial Port"=w435:u32)
              n129 = VISA Read(VISA resource name=w437, byte count=w435, error in (no error)=w436) -> (VISA resource name out=w427:refnum<visa-resource-name>, read buffer=w425:string, error out=w426:errorcluster)  [unwired: 1 out]
            }
          }
        }
        frame "Short DPOS" {
          n130 = case shown="False" w442 {
            tunnel: w444 -> [w450 w465]
            tunnel: w443 -> [w449 w464]
            tunnel: [w448 w462] -> w441
            tunnel: [w447 w463] -> w440
            tunnel: [w446 w461] -> w439
            frame False {
              n131 = Concatenate Strings("BD1_CAT9555_DOUT:30;0" ("write buffer"), "\r\n") -> (w454:string)
              n132 = VISA Write(VISA resource name=w450, write buffer=w454, error in (no error)=w449) -> (VISA resource name out=w459:refnum<visa-resource-name>, error out=w453:errorcluster)  [unwired: 1 out]
              n133 = call "Stall Data Flow.vim"("value in"=w453, "milliseconds to wait"=u32 100) -> ("value out"=w452:errorcluster)  [unwired: 1 out]
              n134 = property class="Instr"(reference=w459, error in=w452) -> (reference out=w458:refnum<visa-resource-name>, error out=w457:errorcluster, "Serial Settings:Number of Bytes at Serial Port"=w456:u32)
              n135 = VISA Read(VISA resource name=w458, byte count=w456, error in (no error)=w457) -> (VISA resource name out=w447:refnum<visa-resource-name>, read buffer=w446:string, error out=w448:errorcluster)  [unwired: 1 out]
            }
            frame True {
              n136 = Concatenate Strings("BD1_CAT9555_DOUT:30;1" ("write buffer"), "\r\n") -> (w469:string)
              n137 = VISA Write(VISA resource name=w465, write buffer=w469, error in (no error)=w464) -> (VISA resource name out=w474:refnum<visa-resource-name>, error out=w468:errorcluster)  [unwired: 1 out]
              n138 = call "Stall Data Flow.vim"("value in"=w468, "milliseconds to wait"=u32 100) -> ("value out"=w467:errorcluster)  [unwired: 1 out]
              n139 = property class="Instr"(reference=w474, error in=w467) -> (reference out=w473:refnum<visa-resource-name>, error out=w472:errorcluster, "Serial Settings:Number of Bytes at Serial Port"=w471:u32)
              n140 = VISA Read(VISA resource name=w473, byte count=w471, error in (no error)=w472) -> (VISA resource name out=w463:refnum<visa-resource-name>, read buffer=w461:string, error out=w462:errorcluster)  [unwired: 1 out]
            }
          }
        }
        frame "meas_PSU_1_12V" {
          n141 = case shown="True" w478 {
            tunnel: w480 -> [w486 w501]
            tunnel: w479 -> [w485 w500]
            tunnel: [w484 w498] -> w477
            tunnel: [w483 w499] -> w476
            tunnel: [w482 w497] -> w475
            frame False {
              n142 = Concatenate Strings("BD1_MeasHLSW:1;2;0" ("write buffer"), "\r\n") -> (w490:string)
              n143 = VISA Write(VISA resource name=w486, write buffer=w490, error in (no error)=w485) -> (VISA resource name out=w495:refnum<visa-resource-name>, error out=w489:errorcluster)  [unwired: 1 out]
              n144 = call "Stall Data Flow.vim"("value in"=w489, "milliseconds to wait"=u32 100) -> ("value out"=w488:errorcluster)  [unwired: 1 out]
              n145 = property class="Instr"(reference=w495, error in=w488) -> (reference out=w494:refnum<visa-resource-name>, error out=w493:errorcluster, "Serial Settings:Number of Bytes at Serial Port"=w492:u32)
              n146 = VISA Read(VISA resource name=w494, byte count=w492, error in (no error)=w493) -> (VISA resource name out=w483:refnum<visa-resource-name>, read buffer=w482:string, error out=w484:errorcluster)  [unwired: 1 out]
            }
            frame True {
              n147 = Concatenate Strings("BD1_MeasHLSW:1;2;1" ("write buffer"), "\r\n") -> (w505:string)
              n148 = VISA Write(VISA resource name=w501, write buffer=w505, error in (no error)=w500) -> (VISA resource name out=w510:refnum<visa-resource-name>, error out=w504:errorcluster)  [unwired: 1 out]
              n149 = call "Stall Data Flow.vim"("value in"=w504, "milliseconds to wait"=u32 100) -> ("value out"=w503:errorcluster)  [unwired: 1 out]
              n150 = property class="Instr"(reference=w510, error in=w503) -> (reference out=w509:refnum<visa-resource-name>, error out=w508:errorcluster, "Serial Settings:Number of Bytes at Serial Port"=w507:u32)
              n151 = VISA Read(VISA resource name=w509, byte count=w507, error in (no error)=w508) -> (VISA resource name out=w499:refnum<visa-resource-name>, read buffer=w497:string, error out=w498:errorcluster)  [unwired: 1 out]
            }
          }
        }
        frame "meas_PSU_2_12V" {
          n152 = case shown="False" w514 {
            tunnel: w516 -> [w522 w537]
            tunnel: w515 -> [w521 w536]
            tunnel: [w520 w534] -> w513
            tunnel: [w519 w535] -> w512
            tunnel: [w518 w533] -> w511
            frame False {
              n153 = Concatenate Strings("BD1_MeasHLSW:3;4;0" ("write buffer"), "\r\n") -> (w526:string)
              n154 = VISA Write(VISA resource name=w522, write buffer=w526, error in (no error)=w521) -> (VISA resource name out=w531:refnum<visa-resource-name>, error out=w525:errorcluster)  [unwired: 1 out]
              n155 = call "Stall Data Flow.vim"("value in"=w525, "milliseconds to wait"=u32 100) -> ("value out"=w524:errorcluster)  [unwired: 1 out]
              n156 = property class="Instr"(reference=w531, error in=w524) -> (reference out=w530:refnum<visa-resource-name>, error out=w529:errorcluster, "Serial Settings:Number of Bytes at Serial Port"=w528:u32)
              n157 = VISA Read(VISA resource name=w530, byte count=w528, error in (no error)=w529) -> (VISA resource name out=w519:refnum<visa-resource-name>, read buffer=w518:string, error out=w520:errorcluster)  [unwired: 1 out]
            }
            frame True {
              n158 = Concatenate Strings("BD1_MeasHLSW:3;4;1" ("write buffer"), "\r\n") -> (w541:string)
              n159 = VISA Write(VISA resource name=w537, write buffer=w541, error in (no error)=w536) -> (VISA resource name out=w546:refnum<visa-resource-name>, error out=w540:errorcluster)  [unwired: 1 out]
              n160 = call "Stall Data Flow.vim"("value in"=w540, "milliseconds to wait"=u32 100) -> ("value out"=w539:errorcluster)  [unwired: 1 out]
              n161 = property class="Instr"(reference=w546, error in=w539) -> (reference out=w545:refnum<visa-resource-name>, error out=w544:errorcluster, "Serial Settings:Number of Bytes at Serial Port"=w543:u32)
              n162 = VISA Read(VISA resource name=w545, byte count=w543, error in (no error)=w544) -> (VISA resource name out=w535:refnum<visa-resource-name>, read buffer=w533:string, error out=w534:errorcluster)  [unwired: 1 out]
            }
          }
        }
        frame "meas_PSU_3_12V" {
          n163 = case shown="False" w550 {
            tunnel: w552 -> [w558 w573]
            tunnel: w551 -> [w557 w572]
            tunnel: [w556 w570] -> w549
            tunnel: [w555 w571] -> w548
            tunnel: [w554 w569] -> w547
            frame False {
              n164 = Concatenate Strings("BD1_MeasHLSW:5;6;0" ("write buffer"), "\r\n") -> (w562:string)
              n165 = VISA Write(VISA resource name=w558, write buffer=w562, error in (no error)=w557) -> (VISA resource name out=w567:refnum<visa-resource-name>, error out=w561:errorcluster)  [unwired: 1 out]
              n166 = call "Stall Data Flow.vim"("value in"=w561, "milliseconds to wait"=u32 100) -> ("value out"=w560:errorcluster)  [unwired: 1 out]
              n167 = property class="Instr"(reference=w567, error in=w560) -> (reference out=w566:refnum<visa-resource-name>, error out=w565:errorcluster, "Serial Settings:Number of Bytes at Serial Port"=w564:u32)
              n168 = VISA Read(VISA resource name=w566, byte count=w564, error in (no error)=w565) -> (VISA resource name out=w555:refnum<visa-resource-name>, read buffer=w554:string, error out=w556:errorcluster)  [unwired: 1 out]
            }
            frame True {
              n169 = Concatenate Strings("BD1_MeasHLSW:5;6;1" ("write buffer"), "\r\n") -> (w577:string)
              n170 = VISA Write(VISA resource name=w573, write buffer=w577, error in (no error)=w572) -> (VISA resource name out=w582:refnum<visa-resource-name>, error out=w576:errorcluster)  [unwired: 1 out]
              n171 = call "Stall Data Flow.vim"("value in"=w576, "milliseconds to wait"=u32 100) -> ("value out"=w575:errorcluster)  [unwired: 1 out]
              n172 = property class="Instr"(reference=w582, error in=w575) -> (reference out=w581:refnum<visa-resource-name>, error out=w580:errorcluster, "Serial Settings:Number of Bytes at Serial Port"=w579:u32)
              n173 = VISA Read(VISA resource name=w581, byte count=w579, error in (no error)=w580) -> (VISA resource name out=w571:refnum<visa-resource-name>, read buffer=w569:string, error out=w570:errorcluster)  [unwired: 1 out]
            }
          }
        }
        frame "meas_UUT_APOS_voltage" {
          n174 = case shown="False" w586 {
            tunnel: w588 -> [w594 w609]
            tunnel: w587 -> [w593 w608]
            tunnel: [w592 w606] -> w585
            tunnel: [w591 w607] -> w584
            tunnel: [w590 w605] -> w583
            frame False {
              n175 = Concatenate Strings("BD1_MeasHLSW:7;8;0" ("write buffer"), "\r\n") -> (w598:string)
              n176 = VISA Write(VISA resource name=w594, write buffer=w598, error in (no error)=w593) -> (VISA resource name out=w603:refnum<visa-resource-name>, error out=w597:errorcluster)  [unwired: 1 out]
              n177 = call "Stall Data Flow.vim"("value in"=w597, "milliseconds to wait"=u32 100) -> ("value out"=w596:errorcluster)  [unwired: 1 out]
              n178 = property class="Instr"(reference=w603, error in=w596) -> (reference out=w602:refnum<visa-resource-name>, error out=w601:errorcluster, "Serial Settings:Number of Bytes at Serial Port"=w600:u32)
              n179 = VISA Read(VISA resource name=w602, byte count=w600, error in (no error)=w601) -> (VISA resource name out=w591:refnum<visa-resource-name>, read buffer=w590:string, error out=w592:errorcluster)  [unwired: 1 out]
            }
            frame True {
              n180 = Concatenate Strings("BD1_MeasHLSW:7;8;1" ("write buffer"), "\r\n") -> (w613:string)
              n181 = VISA Write(VISA resource name=w609, write buffer=w613, error in (no error)=w608) -> (VISA resource name out=w618:refnum<visa-resource-name>, error out=w612:errorcluster)  [unwired: 1 out]
              n182 = call "Stall Data Flow.vim"("value in"=w612, "milliseconds to wait"=u32 100) -> ("value out"=w611:errorcluster)  [unwired: 1 out]
              n183 = property class="Instr"(reference=w618, error in=w611) -> (reference out=w617:refnum<visa-resource-name>, error out=w616:errorcluster, "Serial Settings:Number of Bytes at Serial Port"=w615:u32)
              n184 = VISA Read(VISA resource name=w617, byte count=w615, error in (no error)=w616) -> (VISA resource name out=w607:refnum<visa-resource-name>, read buffer=w605:string, error out=w606:errorcluster)  [unwired: 1 out]
            }
          }
        }
        frame "meas_UUT_ANEG_voltage" {
          n185 = case shown="False" w622 {
            tunnel: w624 -> [w630 w645]
            tunnel: w623 -> [w629 w644]
            tunnel: [w628 w642] -> w621
            tunnel: [w627 w643] -> w620
            tunnel: [w626 w641] -> w619
            frame False {
              n186 = Concatenate Strings("BD1_MeasHLSW:9;10;0" ("write buffer"), "\r\n") -> (w634:string)
              n187 = VISA Write(VISA resource name=w630, write buffer=w634, error in (no error)=w629) -> (VISA resource name out=w639:refnum<visa-resource-name>, error out=w633:errorcluster)  [unwired: 1 out]
              n188 = call "Stall Data Flow.vim"("value in"=w633, "milliseconds to wait"=u32 100) -> ("value out"=w632:errorcluster)  [unwired: 1 out]
              n189 = property class="Instr"(reference=w639, error in=w632) -> (reference out=w638:refnum<visa-resource-name>, error out=w637:errorcluster, "Serial Settings:Number of Bytes at Serial Port"=w636:u32)
              n190 = VISA Read(VISA resource name=w638, byte count=w636, error in (no error)=w637) -> (VISA resource name out=w627:refnum<visa-resource-name>, read buffer=w626:string, error out=w628:errorcluster)  [unwired: 1 out]
            }
            frame True {
              n191 = Concatenate Strings("BD1_MeasHLSW:9;10;1" ("write buffer"), "\r\n") -> (w649:string)
              n192 = VISA Write(VISA resource name=w645, write buffer=w649, error in (no error)=w644) -> (VISA resource name out=w654:refnum<visa-resource-name>, error out=w648:errorcluster)  [unwired: 1 out]
              n193 = call "Stall Data Flow.vim"("value in"=w648, "milliseconds to wait"=u32 100) -> ("value out"=w647:errorcluster)  [unwired: 1 out]
              n194 = property class="Instr"(reference=w654, error in=w647) -> (reference out=w653:refnum<visa-resource-name>, error out=w652:errorcluster, "Serial Settings:Number of Bytes at Serial Port"=w651:u32)
              n195 = VISA Read(VISA resource name=w653, byte count=w651, error in (no error)=w652) -> (VISA resource name out=w643:refnum<visa-resource-name>, read buffer=w641:string, error out=w642:errorcluster)  [unwired: 1 out]
            }
          }
        }
        frame "meas_UUT_DPOS_voltage" {
          n196 = case shown="True" w658 {
            tunnel: w660 -> [w666 w681]
            tunnel: w659 -> [w665 w680]
            tunnel: [w664 w678] -> w657
            tunnel: [w663 w679] -> w656
            tunnel: [w662 w677] -> w655
            frame False {
              n197 = Concatenate Strings("BD1_MeasHLSW:11;12;0" ("write buffer"), "\r\n") -> (w670:string)
              n198 = VISA Write(VISA resource name=w666, write buffer=w670, error in (no error)=w665) -> (VISA resource name out=w675:refnum<visa-resource-name>, error out=w669:errorcluster)  [unwired: 1 out]
              n199 = call "Stall Data Flow.vim"("value in"=w669, "milliseconds to wait"=u32 100) -> ("value out"=w668:errorcluster)  [unwired: 1 out]
              n200 = property class="Instr"(reference=w675, error in=w668) -> (reference out=w674:refnum<visa-resource-name>, error out=w673:errorcluster, "Serial Settings:Number of Bytes at Serial Port"=w672:u32)
              n201 = VISA Read(VISA resource name=w674, byte count=w672, error in (no error)=w673) -> (VISA resource name out=w663:refnum<visa-resource-name>, read buffer=w662:string, error out=w664:errorcluster)  [unwired: 1 out]
            }
            frame True {
              n202 = Concatenate Strings("BD1_MeasHLSW:11;12;1" ("write buffer"), "\r\n") -> (w685:string)
              n203 = VISA Write(VISA resource name=w681, write buffer=w685, error in (no error)=w680) -> (VISA resource name out=w690:refnum<visa-resource-name>, error out=w684:errorcluster)  [unwired: 1 out]
              n204 = call "Stall Data Flow.vim"("value in"=w684, "milliseconds to wait"=u32 100) -> ("value out"=w683:errorcluster)  [unwired: 1 out]
              n205 = property class="Instr"(reference=w690, error in=w683) -> (reference out=w689:refnum<visa-resource-name>, error out=w688:errorcluster, "Serial Settings:Number of Bytes at Serial Port"=w687:u32)
              n206 = VISA Read(VISA resource name=w689, byte count=w687, error in (no error)=w688) -> (VISA resource name out=w679:refnum<visa-resource-name>, read buffer=w677:string, error out=w678:errorcluster)  [unwired: 1 out]
            }
          }
        }
        frame "meas_LOAD_APOS_voltage" {
          n207 = case shown="False" w694 {
            tunnel: w696 -> [w702 w717]
            tunnel: w695 -> [w701 w716]
            tunnel: [w700 w714] -> w693
            tunnel: [w699 w715] -> w692
            tunnel: [w698 w713] -> w691
            frame False {
              n208 = Concatenate Strings("BD1_MeasHLSW:13;14;0" ("write buffer"), "\r\n") -> (w706:string)
              n209 = VISA Write(VISA resource name=w702, write buffer=w706, error in (no error)=w701) -> (VISA resource name out=w711:refnum<visa-resource-name>, error out=w705:errorcluster)  [unwired: 1 out]
              n210 = call "Stall Data Flow.vim"("value in"=w705, "milliseconds to wait"=u32 100) -> ("value out"=w704:errorcluster)  [unwired: 1 out]
              n211 = property class="Instr"(reference=w711, error in=w704) -> (reference out=w710:refnum<visa-resource-name>, error out=w709:errorcluster, "Serial Settings:Number of Bytes at Serial Port"=w708:u32)
              n212 = VISA Read(VISA resource name=w710, byte count=w708, error in (no error)=w709) -> (VISA resource name out=w699:refnum<visa-resource-name>, read buffer=w698:string, error out=w700:errorcluster)  [unwired: 1 out]
            }
            frame True {
              n213 = Concatenate Strings("BD1_MeasHLSW:13;14;1" ("write buffer"), "\r\n") -> (w721:string)
              n214 = VISA Write(VISA resource name=w717, write buffer=w721, error in (no error)=w716) -> (VISA resource name out=w726:refnum<visa-resource-name>, error out=w720:errorcluster)  [unwired: 1 out]
              n215 = call "Stall Data Flow.vim"("value in"=w720, "milliseconds to wait"=u32 100) -> ("value out"=w719:errorcluster)  [unwired: 1 out]
              n216 = property class="Instr"(reference=w726, error in=w719) -> (reference out=w725:refnum<visa-resource-name>, error out=w724:errorcluster, "Serial Settings:Number of Bytes at Serial Port"=w723:u32)
              n217 = VISA Read(VISA resource name=w725, byte count=w723, error in (no error)=w724) -> (VISA resource name out=w715:refnum<visa-resource-name>, read buffer=w713:string, error out=w714:errorcluster)  [unwired: 1 out]
            }
          }
        }
        frame "meas_LOAD_ANEG_voltage" {
          n218 = case shown="False" w730 {
            tunnel: w732 -> [w738 w753]
            tunnel: w731 -> [w737 w752]
            tunnel: [w736 w750] -> w729
            tunnel: [w735 w751] -> w728
            tunnel: [w734 w749] -> w727
            frame False {
              n219 = Concatenate Strings("BD1_MeasHLSW:15;16;0" ("write buffer"), "\r\n") -> (w742:string)
              n220 = VISA Write(VISA resource name=w738, write buffer=w742, error in (no error)=w737) -> (VISA resource name out=w747:refnum<visa-resource-name>, error out=w741:errorcluster)  [unwired: 1 out]
              n221 = call "Stall Data Flow.vim"("value in"=w741, "milliseconds to wait"=u32 100) -> ("value out"=w740:errorcluster)  [unwired: 1 out]
              n222 = property class="Instr"(reference=w747, error in=w740) -> (reference out=w746:refnum<visa-resource-name>, error out=w745:errorcluster, "Serial Settings:Number of Bytes at Serial Port"=w744:u32)
              n223 = VISA Read(VISA resource name=w746, byte count=w744, error in (no error)=w745) -> (VISA resource name out=w735:refnum<visa-resource-name>, read buffer=w734:string, error out=w736:errorcluster)  [unwired: 1 out]
            }
            frame True {
              n224 = Concatenate Strings("BD1_MeasHLSW:15;16;1" ("write buffer"), "\r\n") -> (w757:string)
              n225 = VISA Write(VISA resource name=w753, write buffer=w757, error in (no error)=w752) -> (VISA resource name out=w762:refnum<visa-resource-name>, error out=w756:errorcluster)  [unwired: 1 out]
              n226 = call "Stall Data Flow.vim"("value in"=w756, "milliseconds to wait"=u32 100) -> ("value out"=w755:errorcluster)  [unwired: 1 out]
              n227 = property class="Instr"(reference=w762, error in=w755) -> (reference out=w761:refnum<visa-resource-name>, error out=w760:errorcluster, "Serial Settings:Number of Bytes at Serial Port"=w759:u32)
              n228 = VISA Read(VISA resource name=w761, byte count=w759, error in (no error)=w760) -> (VISA resource name out=w751:refnum<visa-resource-name>, read buffer=w749:string, error out=w750:errorcluster)  [unwired: 1 out]
            }
          }
        }
        frame "meas_LOAD_DPOS_voltage" {
          n229 = case shown="False" w766 {
            tunnel: w768 -> [w774 w789]
            tunnel: w767 -> [w773 w788]
            tunnel: [w772 w786] -> w765
            tunnel: [w771 w787] -> w764
            tunnel: [w770 w785] -> w763
            frame False {
              n230 = Concatenate Strings("BD1_MeasHLSW:17;18;0" ("write buffer"), "\r\n") -> (w778:string)
              n231 = VISA Write(VISA resource name=w774, write buffer=w778, error in (no error)=w773) -> (VISA resource name out=w783:refnum<visa-resource-name>, error out=w777:errorcluster)  [unwired: 1 out]
              n232 = call "Stall Data Flow.vim"("value in"=w777, "milliseconds to wait"=u32 100) -> ("value out"=w776:errorcluster)  [unwired: 1 out]
              n233 = property class="Instr"(reference=w783, error in=w776) -> (reference out=w782:refnum<visa-resource-name>, error out=w781:errorcluster, "Serial Settings:Number of Bytes at Serial Port"=w780:u32)
              n234 = VISA Read(VISA resource name=w782, byte count=w780, error in (no error)=w781) -> (VISA resource name out=w771:refnum<visa-resource-name>, read buffer=w770:string, error out=w772:errorcluster)  [unwired: 1 out]
            }
            frame True {
              n235 = Concatenate Strings("BD1_MeasHLSW:17;18;1" ("write buffer"), "\r\n") -> (w793:string)
              n236 = VISA Write(VISA resource name=w789, write buffer=w793, error in (no error)=w788) -> (VISA resource name out=w798:refnum<visa-resource-name>, error out=w792:errorcluster)  [unwired: 1 out]
              n237 = call "Stall Data Flow.vim"("value in"=w792, "milliseconds to wait"=u32 100) -> ("value out"=w791:errorcluster)  [unwired: 1 out]
              n238 = property class="Instr"(reference=w798, error in=w791) -> (reference out=w797:refnum<visa-resource-name>, error out=w796:errorcluster, "Serial Settings:Number of Bytes at Serial Port"=w795:u32)
              n239 = VISA Read(VISA resource name=w797, byte count=w795, error in (no error)=w796) -> (VISA resource name out=w787:refnum<visa-resource-name>, read buffer=w785:string, error out=w786:errorcluster)  [unwired: 1 out]
            }
          }
        }
        frame "UUT_FCT_power_SW" {
          n240 = case shown="False" w802 {
            tunnel: w804 -> [w810 w825]
            tunnel: w803 -> [w809 w824]
            tunnel: [w808 w822] -> w801
            tunnel: [w807 w823] -> w800
            tunnel: [w806 w821] -> w799
            frame False {
              n241 = Concatenate Strings("BD2_CAT9555_DOUT:1;0" ("write buffer"), "\r\n") -> (w814:string)
              n242 = VISA Write(VISA resource name=w810, write buffer=w814, error in (no error)=w809) -> (VISA resource name out=w819:refnum<visa-resource-name>, error out=w813:errorcluster)  [unwired: 1 out]
              n243 = call "Stall Data Flow.vim"("value in"=w813, "milliseconds to wait"=u32 100) -> ("value out"=w812:errorcluster)  [unwired: 1 out]
              n244 = property class="Instr"(reference=w819, error in=w812) -> (reference out=w818:refnum<visa-resource-name>, error out=w817:errorcluster, "Serial Settings:Number of Bytes at Serial Port"=w816:u32)
              n245 = VISA Read(VISA resource name=w818, byte count=w816, error in (no error)=w817) -> (VISA resource name out=w807:refnum<visa-resource-name>, read buffer=w806:string, error out=w808:errorcluster)  [unwired: 1 out]
            }
            frame True {
              n246 = Concatenate Strings("BD2_CAT9555_DOUT:1;1" ("write buffer"), "\r\n") -> (w829:string)
              n247 = VISA Write(VISA resource name=w825, write buffer=w829, error in (no error)=w824) -> (VISA resource name out=w834:refnum<visa-resource-name>, error out=w828:errorcluster)  [unwired: 1 out]
              n248 = call "Stall Data Flow.vim"("value in"=w828, "milliseconds to wait"=u32 100) -> ("value out"=w827:errorcluster)  [unwired: 1 out]
              n249 = property class="Instr"(reference=w834, error in=w827) -> (reference out=w833:refnum<visa-resource-name>, error out=w832:errorcluster, "Serial Settings:Number of Bytes at Serial Port"=w831:u32)
              n250 = VISA Read(VISA resource name=w833, byte count=w831, error in (no error)=w832) -> (VISA resource name out=w823:refnum<visa-resource-name>, read buffer=w821:string, error out=w822:errorcluster)  [unwired: 1 out]
            }
          }
        }
        frame "FCT_FAN_SW" {
          n251 = case shown="False" w838 {
            tunnel: w840 -> [w846 w861]
            tunnel: w839 -> [w845 w860]
            tunnel: [w844 w858] -> w837
            tunnel: [w843 w859] -> w836
            tunnel: [w842 w857] -> w835
            frame False {
              n252 = Concatenate Strings("BD2_CAT9555_DOUT:5;0" ("write buffer"), "\r\n") -> (w850:string)
              n253 = VISA Write(VISA resource name=w846, write buffer=w850, error in (no error)=w845) -> (VISA resource name out=w855:refnum<visa-resource-name>, error out=w849:errorcluster)  [unwired: 1 out]
              n254 = call "Stall Data Flow.vim"("value in"=w849, "milliseconds to wait"=u32 100) -> ("value out"=w848:errorcluster)  [unwired: 1 out]
              n255 = property class="Instr"(reference=w855, error in=w848) -> (reference out=w854:refnum<visa-resource-name>, error out=w853:errorcluster, "Serial Settings:Number of Bytes at Serial Port"=w852:u32)
              n256 = VISA Read(VISA resource name=w854, byte count=w852, error in (no error)=w853) -> (VISA resource name out=w843:refnum<visa-resource-name>, read buffer=w842:string, error out=w844:errorcluster)  [unwired: 1 out]
            }
            frame True {
              n257 = Concatenate Strings("BD2_CAT9555_DOUT:5;1" ("write buffer"), "\r\n") -> (w865:string)
              n258 = VISA Write(VISA resource name=w861, write buffer=w865, error in (no error)=w860) -> (VISA resource name out=w870:refnum<visa-resource-name>, error out=w864:errorcluster)  [unwired: 1 out]
              n259 = call "Stall Data Flow.vim"("value in"=w864, "milliseconds to wait"=u32 100) -> ("value out"=w863:errorcluster)  [unwired: 1 out]
              n260 = property class="Instr"(reference=w870, error in=w863) -> (reference out=w869:refnum<visa-resource-name>, error out=w868:errorcluster, "Serial Settings:Number of Bytes at Serial Port"=w867:u32)
              n261 = VISA Read(VISA resource name=w869, byte count=w867, error in (no error)=w868) -> (VISA resource name out=w859:refnum<visa-resource-name>, read buffer=w857:string, error out=w858:errorcluster)  [unwired: 1 out]
            }
          }
        }
        frame "Burn_in_FAN_SW" {
          n262 = case shown="True" w874 {
            tunnel: w876 -> [w882 w897]
            tunnel: w875 -> [w881 w896]
            tunnel: [w880 w894] -> w871
            tunnel: [w879 w895] -> w872
            tunnel: [w878 w893] -> w873
            frame False {
              n263 = Concatenate Strings("BD2_CAT9555_DOUT:6;0" ("write buffer"), "\r\n") -> (w886:string)
              n264 = VISA Write(VISA resource name=w882, write buffer=w886, error in (no error)=w881) -> (VISA resource name out=w891:refnum<visa-resource-name>, error out=w885:errorcluster)  [unwired: 1 out]
              n265 = call "Stall Data Flow.vim"("value in"=w885, "milliseconds to wait"=u32 100) -> ("value out"=w884:errorcluster)  [unwired: 1 out]
              n266 = property class="Instr"(reference=w891, error in=w884) -> (reference out=w890:refnum<visa-resource-name>, error out=w889:errorcluster, "Serial Settings:Number of Bytes at Serial Port"=w888:u32)
              n267 = VISA Read(VISA resource name=w890, byte count=w888, error in (no error)=w889) -> (VISA resource name out=w879:refnum<visa-resource-name>, read buffer=w878:string, error out=w880:errorcluster)  [unwired: 1 out]
            }
            frame True {
              n268 = Concatenate Strings("BD2_CAT9555_DOUT:6;1" ("write buffer"), "\r\n") -> (w901:string)
              n269 = VISA Write(VISA resource name=w897, write buffer=w901, error in (no error)=w896) -> (VISA resource name out=w906:refnum<visa-resource-name>, error out=w900:errorcluster)  [unwired: 1 out]
              n270 = call "Stall Data Flow.vim"("value in"=w900, "milliseconds to wait"=u32 100) -> ("value out"=w899:errorcluster)  [unwired: 1 out]
              n271 = property class="Instr"(reference=w906, error in=w899) -> (reference out=w905:refnum<visa-resource-name>, error out=w904:errorcluster, "Serial Settings:Number of Bytes at Serial Port"=w903:u32)
              n272 = VISA Read(VISA resource name=w905, byte count=w903, error in (no error)=w904) -> (VISA resource name out=w895:refnum<visa-resource-name>, read buffer=w893:string, error out=w894:errorcluster)  [unwired: 1 out]
            }
          }
        }
        frame "FCT_24V_SW" {
          n273 = case shown="False" w910 {
            tunnel: w912 -> [w918 w933]
            tunnel: w911 -> [w917 w932]
            tunnel: [w916 w930] -> w909
            tunnel: [w915 w931] -> w908
            tunnel: [w914 w929] -> w907
            frame False {
              n274 = Concatenate Strings("BD2_CAT9555_DOUT:7;0" ("write buffer"), "\r\n") -> (w922:string)
              n275 = VISA Write(VISA resource name=w918, write buffer=w922, error in (no error)=w917) -> (VISA resource name out=w927:refnum<visa-resource-name>, error out=w921:errorcluster)  [unwired: 1 out]
              n276 = call "Stall Data Flow.vim"("value in"=w921, "milliseconds to wait"=u32 100) -> ("value out"=w920:errorcluster)  [unwired: 1 out]
              n277 = property class="Instr"(reference=w927, error in=w920) -> (reference out=w926:refnum<visa-resource-name>, error out=w925:errorcluster, "Serial Settings:Number of Bytes at Serial Port"=w924:u32)
              n278 = VISA Read(VISA resource name=w926, byte count=w924, error in (no error)=w925) -> (VISA resource name out=w915:refnum<visa-resource-name>, read buffer=w914:string, error out=w916:errorcluster)  [unwired: 1 out]
            }
            frame True {
              n279 = Concatenate Strings("BD2_CAT9555_DOUT:7;1" ("write buffer"), "\r\n") -> (w937:string)
              n280 = VISA Write(VISA resource name=w933, write buffer=w937, error in (no error)=w932) -> (VISA resource name out=w942:refnum<visa-resource-name>, error out=w936:errorcluster)  [unwired: 1 out]
              n281 = call "Stall Data Flow.vim"("value in"=w936, "milliseconds to wait"=u32 100) -> ("value out"=w935:errorcluster)  [unwired: 1 out]
              n282 = property class="Instr"(reference=w942, error in=w935) -> (reference out=w941:refnum<visa-resource-name>, error out=w940:errorcluster, "Serial Settings:Number of Bytes at Serial Port"=w939:u32)
              n283 = VISA Read(VISA resource name=w941, byte count=w939, error in (no error)=w940) -> (VISA resource name out=w931:refnum<visa-resource-name>, read buffer=w929:string, error out=w930:errorcluster)  [unwired: 1 out]
            }
          }
        }
        frame "DMM_SW" {
          n284 = case shown="True" w946 {
            tunnel: w948 -> [w954 w974]
            tunnel: w947 -> [w953 w973]
            tunnel: [w952 w971] -> w945
            tunnel: [w951 w972] -> w944
            tunnel: [w950 w970] -> w943
            frame False {
              n285 = for {
                tunnel: string[] ["BD1_TestBusOFF", "BD2_TestBusOFF"] -> [w964] mode=indexing
                shift-right: [w968] -> w961
                shift-left: w954 -> [w966]
                shift-right: [w967] -> w957
                shift-left: w953 -> [w965]
                n286 = Concatenate Strings(w964, "\r\n") -> (w963:string)
                n287 = VISA Write(VISA resource name=w966, write buffer=w963, error in (no error)=w965) -> (VISA resource name out=w968:refnum<visa-resource-name>, error out=w967:errorcluster)  [unwired: 1 out]
              }
              n288 = call "Stall Data Flow.vim"("value in"=w957, "milliseconds to wait"=u32 100) -> ("value out"=w956:errorcluster)  [unwired: 1 out]
              n289 = property class="Instr"(reference=w961, error in=w956) -> (reference out=w960:refnum<visa-resource-name>, error out=w959:errorcluster, "Serial Settings:Number of Bytes at Serial Port"=w958:u32)
              n290 = VISA Read(VISA resource name=w960, byte count=w958, error in (no error)=w959) -> (VISA resource name out=w951:refnum<visa-resource-name>, read buffer=w950:string, error out=w952:errorcluster)  [unwired: 1 out]
            }
            frame True {
              n291 = for {
                tunnel: string[] ["BD1_TestBusON", "BD2_TestBusON"] -> [w984] mode=indexing
                shift-right: [w988] -> w981
                shift-left: w974 -> [w986]
                shift-right: [w987] -> w977
                shift-left: w973 -> [w985]
                n292 = Concatenate Strings(w984, "\r\n") -> (w982:string)
                n293 = VISA Write(VISA resource name=w986, write buffer=w982, error in (no error)=w985) -> (VISA resource name out=w988:refnum<visa-resource-name>, error out=w987:errorcluster)  [unwired: 1 out]
              }
              n294 = call "Stall Data Flow.vim"("value in"=w977, "milliseconds to wait"=u32 100) -> ("value out"=w976:errorcluster)  [unwired: 1 out]
              n295 = property class="Instr"(reference=w981, error in=w976) -> (reference out=w980:refnum<visa-resource-name>, error out=w979:errorcluster, "Serial Settings:Number of Bytes at Serial Port"=w978:u32)
              n296 = VISA Read(VISA resource name=w980, byte count=w978, error in (no error)=w979) -> (VISA resource name out=w972:refnum<visa-resource-name>, read buffer=w970:string, error out=w971:errorcluster)  [unwired: 1 out]
            }
          }
        }
        frame "USB_Reset" {
          n297 = case shown="False" w992 {
            tunnel: w993 -> [w1000 w1015]
            tunnel: w994 -> [w999 w1014]
            tunnel: [w998 w1012] -> w991
            tunnel: [w997 w1013] -> w990
            tunnel: [w996 w1011] -> w989
            frame False {
              n298 = Concatenate Strings("BD2_CAT9555_DOUT:9;0" ("write buffer"), "\r\n") -> (w1004:string)
              n299 = VISA Write(VISA resource name=w1000, write buffer=w1004, error in (no error)=w999) -> (VISA resource name out=w1009:refnum<visa-resource-name>, error out=w1003:errorcluster)  [unwired: 1 out]
              n300 = call "Stall Data Flow.vim"("value in"=w1003, "milliseconds to wait"=u32 100) -> ("value out"=w1002:errorcluster)  [unwired: 1 out]
              n301 = property class="Instr"(reference=w1009, error in=w1002) -> (reference out=w1008:refnum<visa-resource-name>, error out=w1007:errorcluster, "Serial Settings:Number of Bytes at Serial Port"=w1006:u32)
              n302 = VISA Read(VISA resource name=w1008, byte count=w1006, error in (no error)=w1007) -> (VISA resource name out=w997:refnum<visa-resource-name>, read buffer=w996:string, error out=w998:errorcluster)  [unwired: 1 out]
            }
            frame True {
              n303 = Concatenate Strings("BD2_CAT9555_DOUT:9;1" ("write buffer"), "\r\n") -> (w1019:string)
              n304 = VISA Write(VISA resource name=w1015, write buffer=w1019, error in (no error)=w1014) -> (VISA resource name out=w1024:refnum<visa-resource-name>, error out=w1018:errorcluster)  [unwired: 1 out]
              n305 = call "Stall Data Flow.vim"("value in"=w1018, "milliseconds to wait"=u32 100) -> ("value out"=w1017:errorcluster)  [unwired: 1 out]
              n306 = property class="Instr"(reference=w1024, error in=w1017) -> (reference out=w1023:refnum<visa-resource-name>, error out=w1022:errorcluster, "Serial Settings:Number of Bytes at Serial Port"=w1021:u32)
              n307 = VISA Read(VISA resource name=w1023, byte count=w1021, error in (no error)=w1022) -> (VISA resource name out=w1013:refnum<visa-resource-name>, read buffer=w1011:string, error out=w1012:errorcluster)  [unwired: 1 out]
            }
          }
        }
      }
      n308 = VISA Close(VISA resource name=w20, error in (no error)=w21) -> (error out=w14:errorcluster)
      n309 = Search and Replace String(input string=w19, search string="Succefull") -> (number of replacements=w17:i32)  [unwired: 6 in, 3 out]
      n310 = call <vilib>:"Clear Errors.vi"("error in (no error)"=w14, "specific error code to clear (0: all)"=1073676294) -> ("error out"=w11:errorcluster)  [unwired: 4 in, 1 out]
      n311 = Greater?(x=w17, y=0) -> (0:w12:bool)
      n312 = Select(t=w11, s=w12, f=errorcluster {"status"=TRUE, "code"=5000, "source"="testbox return error"}) -> (s? t:f=w10:errorcluster)
    }
    frame Error {
    }
  }
  "VISA resource out" <- w4
  "error out" <- w1
  "read buffer" <- w3
  "Result" <- w2
